vi "FTW-Publisher-Destroy.vi"(0 "FTW-Publisher In":refnum<class "FTW-Publisher.lvclass">, 11 "error in":errorcluster) -> (15 "error out":errorcluster)   [LabVIEW 2013, in "FTW-Publisher.lvclass"]
uses:
  FTW-Publisher.lvclass
  <vilib>/event_ctls.llb/usereventprio.ctl
  Message/Base/FTW-Message.lvclass
  FTW-Publisher.lvclass/FTW-Publisher.ctl
  Listener/FTW-Listener.lvclass
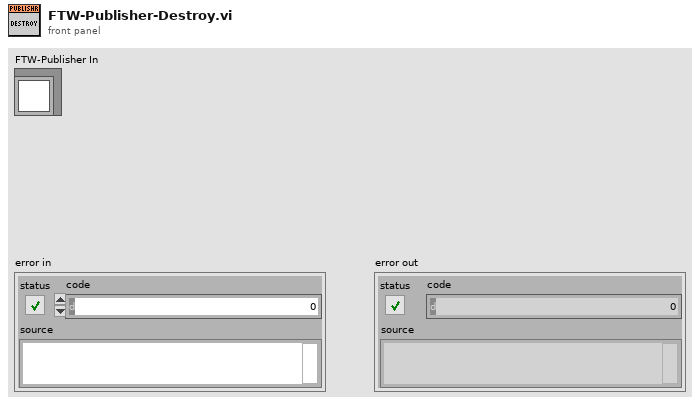
[diagram p1: front panel]
types:
  T1 = typedef "usereventprio.ctl" = enum32{"high priority", "normal priority"}
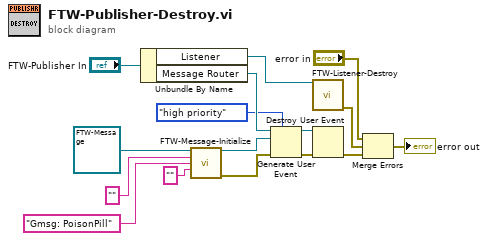
[diagram p0: block diagram]
diagram:
  n1 = Unbundle By Name("FTW-Publisher In") -> ("Listener"=w12:refnum<class "FTW-Listener.lvclass">, "Message Router"=w13:refnum<user-event>)
  n2 = call-dynamic "FTW-Message-Initialize.vi"("FTW Message"=refnum<class "FTW-Message.lvclass"> refnum, "Sender Identity"="", "Message Header"="Gmsg: PoisonPill", "Message Body"="") -> ("FTW Message out"=w6:refnum<class "FTW-Message.lvclass">, "error out"=w5:errorcluster)  [unwired: 10 in]
  n3 = Generate User Event(priority (normal)=usereventprio."high priority", user event=w13, event data cluster=w6, error in=w5) -> (user event out=w9:refnum<user-event>, error out=w8:errorcluster)
  n4 = call-dynamic "FTW-Listener-Destroy.vi"("Gmsg_Listener In"=w12) -> ("error out"=w11:errorcluster)  [unwired: 14 in]
  n5 = Destroy User Event(user event=w9, error in=w8) -> (error out=w10:errorcluster)
  n6 = Merge Errors("error in", w11, w10) -> (→"error out":errorcluster)
